vi "DAQ-node_streamIO.vi"(8 "error in":errorcluster, 10 "Stream Cluster":T1={"Reader IP Addr"="localhost", "Writer Endpoint"="DAQ001", "Reader Endpoint"="CTR001", "Channel Definitions"=[], "Writer Endpoint Ref"="", "Reader Endpoint Ref"="", "steam error"={"status"=FALSE, "code"=0, "source"=""}}, 11 "queue out":refnum<queue>) -> (0 "error out":errorcluster, 3 "Reader URL":string)   [LabVIEW 2024]
uses:
  DAQ-node_streamIO_settings.ctl
  DAQ-node_streamIO_states.ctl
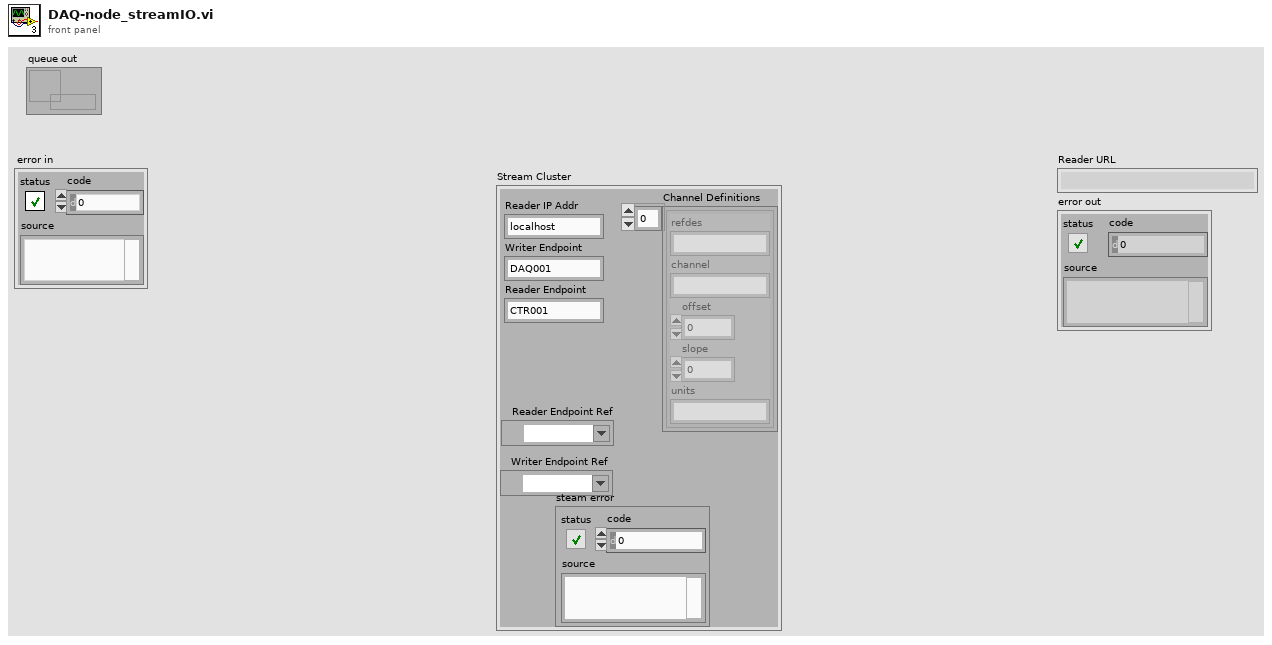
[diagram p1: front panel]
types:
  T1 = typedef "DAQ-node_streamIO_settings.ctl" = cluster{"Reader IP Addr":string, "Writer Endpoint":string, "Reader Endpoint":string, "Channel Definitions":cluster{"refdes":string, "channel":string, "offset":dbl, "slope":dbl, "units":string}[], "Writer Endpoint Ref":refnum<k21>, "Reader Endpoint Ref":refnum<k21>, "steam error":errorcluster}
  T2 = typedef "DAQ-node_streamIO_states.ctl" = enum16{"Fault", "Initilize", "Stream", "Close"}
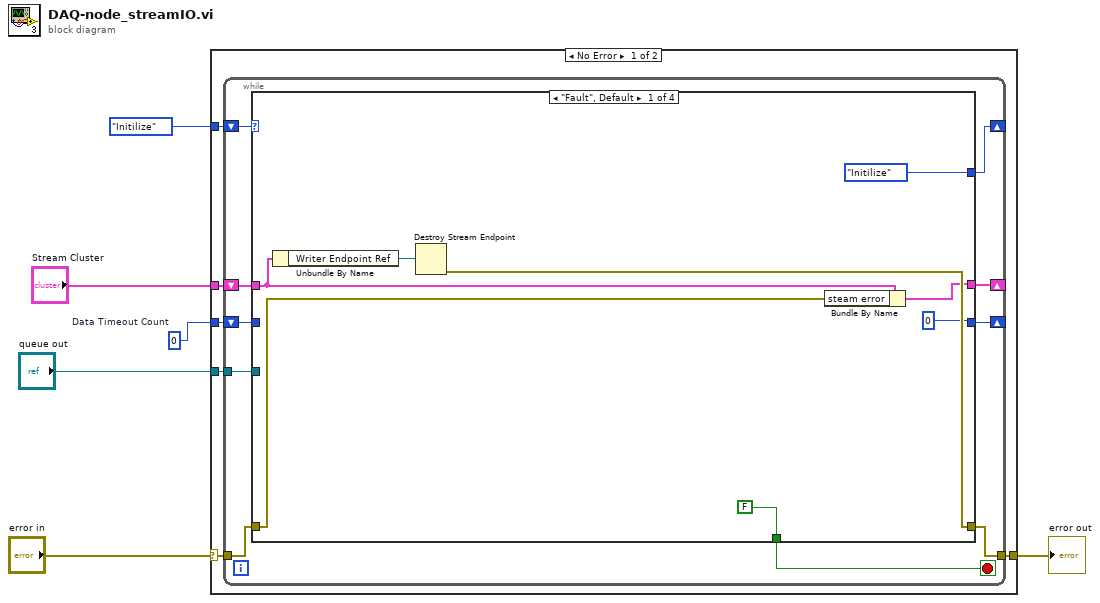
[diagram p0: block diagram]
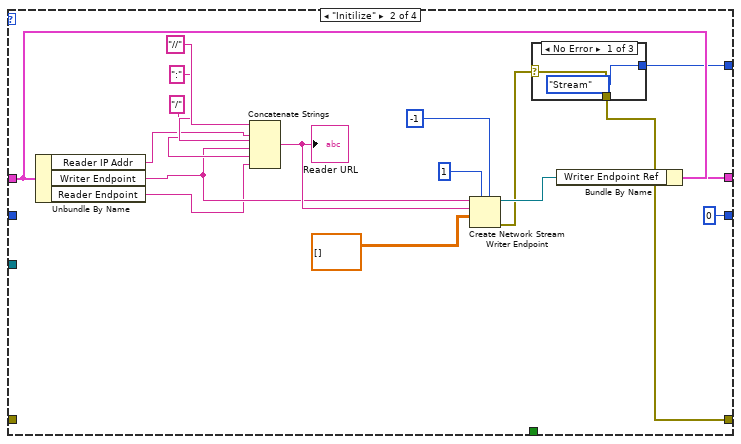
[diagram p2: hidden frame]
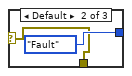
[diagram p3: hidden frame]
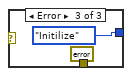
[diagram p4: hidden frame]
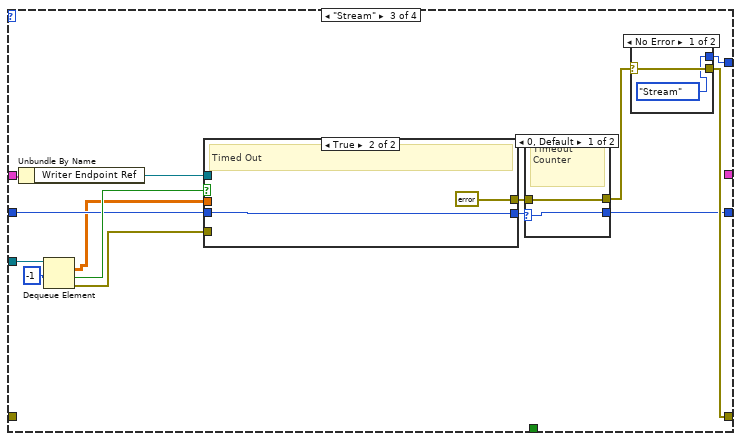
[diagram p5: hidden frame]
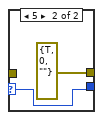
[diagram p6: hidden frame]
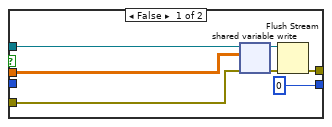
[diagram p7: hidden frame]
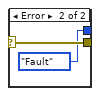
[diagram p8: hidden frame]
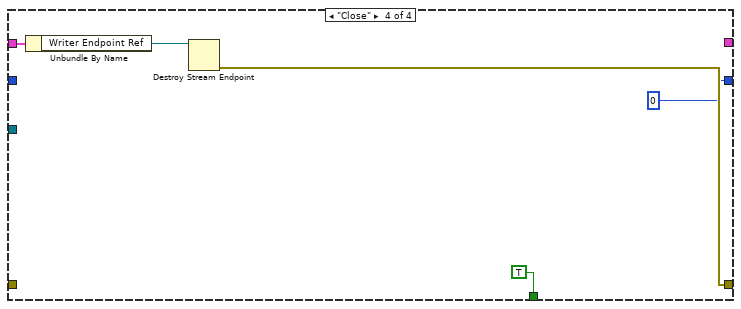
[diagram p9: hidden frame]
diagram:
  w3 = 0  # Data Timeout Count
  n1 = case shown="No Error" "error in" {
    selector: "error in" -> [w9 w90]
    tunnel: [w10 w90] -> w5
    tunnel: DAQ-node_streamIO_states."Initilize" -> [w12 _]
    tunnel: "Stream Cluster" -> [w11 _]
    tunnel: w3 -> [w8 _]
    tunnel: "queue out" -> [w7 _]
    frame No Error {
      n2 = while {
        shift-right: [w16] -> _
        shift-left: w12 -> [w22]
        shift-right: [w19] -> _
        shift-left: w11 -> [w20]
        tunnel: [w18] -> w10
        tunnel: w9 -> [w17]
        shift-right: [w14] -> _
        shift-left: w8 -> [w15]
        tunnel: w7 -> [w13]
        stop <- w21 stop-if-true
        n3 = case shown="\"Fault\", Default" w22 {
          tunnel: [FALSE _ _ TRUE] -> w21
          tunnel: w20 -> [w25 w37 w67 w88]
          tunnel: [w26 w35 _ _] -> w19
          tunnel: [w27 w32 w66 w87] -> w18
          tunnel: w17 -> [w24 _ _ _]
          tunnel: [DAQ-node_streamIO_states."Initilize" w34 w65 _] -> w16
          tunnel: w15 -> [_ _ w61 _]
          tunnel: [0 0 w57 0] -> w14
          tunnel: w13 -> [_ _ w56 _]
          frame "Fault", Default {
            n4 = Unbundle By Name(w25) -> ("Writer Endpoint Ref"=w28:refnum<k21>)
            n5 = Destroy Stream Endpoint(11:w28) -> (0:w27:errorcluster)  [unwired: 1 in]
            n6 = Bundle By Name(cluster=w25, "steam error"=w24) -> (w26:T1)
          }
          frame "Initilize" {
            n7 = Unbundle By Name(w37) -> ("Reader IP Addr"=w40:string, "Writer Endpoint"=w39:string, "Reader Endpoint"=w38:string)
            n8 = Concatenate Strings("//" ("string"), w40, ":" ("string"), w39, "/" ("string"), w38) -> (w47:string)
            "Reader URL" <- w47
            n9 = Create Network Stream Writer Endpoint(5:-1 ("timeout in ms (-1)"), 7:1 ("reader buffer size"), 9:dbl[][] [], 10:w47, 11:w39) -> (0:w33:errorcluster, 3:w36:refnum<k21>)  [unwired: 2 in]
            n10 = case shown="No Error" w33 {
              selector: w33 -> [w48 w50 _]
              tunnel: [DAQ-node_streamIO_states."Stream" DAQ-node_streamIO_states."Fault" DAQ-node_streamIO_states."Initilize"] -> w34
              tunnel: [w48 w50 errorcluster {"status"=FALSE, "code"=0, "source"=""} ("error out")] -> w32
              frame No Error {
              }
              frame Default {
              }
              frame Error {
              }
            }
            n11 = Bundle By Name(cluster=w37, "Writer Endpoint Ref"=w36) -> (w35:T1)
          }
          frame "Stream" {
            n12 = Unbundle By Name(w67) -> ("Writer Endpoint Ref"=w64:refnum<k21>)
            n13 = Dequeue Element(queue=w56, timeout in ms (-1)=-1) -> (element=w55:dbl[][], timed out?=w62:bool, error out=w63:errorcluster)  [unwired: 1 in, 1 out]
            n14 = case shown="True" w62 {
              tunnel: w64 -> [w74 _]
              tunnel: w63 -> [w75 _]
              tunnel: w61 -> [_ w79]
              tunnel: [0 w79] -> w60
              tunnel: [w77 errorcluster {"status"=FALSE, "code"=0, "source"=""} ("error out")] -> w58
              tunnel: w55 -> [w72 _]
              frame False {
                n15 = shared-variable-write(w74, w75, w72) -> (w73:refnum<k21>, w76:errorcluster)  [unwired: 1 in, 1 out]
                n16 = Flush Stream(8:w76, 11:w73) -> (0:w77:errorcluster)  [unwired: 2 in, 2 out]
              }
              frame True {
                # "Timed Out"
              }
            }
            n17 = case shown="0, Default" w60 {
              selector: w60 -> [w68 w70]
              tunnel: [w69 errorcluster {"status"=TRUE, "code"=0, "source"=""} ("error out")] -> w59
              tunnel: w58 -> [w69 _]
              tunnel: [w68 w70] -> w57
              frame 0, Default {
                # "Timeout Counter"
              }
              frame 5 {
              }
            }
            n18 = case shown="No Error" w59 {
              selector: w59 -> [w82 w84]
              tunnel: [w82 w84] -> w66
              tunnel: [DAQ-node_streamIO_states."Stream" DAQ-node_streamIO_states."Fault"] -> w65
              frame No Error {
              }
              frame Error {
              }
            }
          }
          frame "Close" {
            n19 = Unbundle By Name(w88) -> ("Writer Endpoint Ref"=w86:refnum<k21>)
            n20 = Destroy Stream Endpoint(11:w86) -> (0:w87:errorcluster)  [unwired: 1 in]
          }
        }
      }
    }
    frame Error {
    }
  }
  "error out" <- w5
